vi "Write HttpRequestMessage.vi"(8 "error in (no error)":errorcluster, 10 "LabVIEWHTTPClient_NET.lvlib:HttpRequestMessage.lvclass":refnum<class "HttpRequestMessage.lvclass">, 11 "HttpResponseMessage in":refnum<class "HttpResponseMessage.lvclass">) -> (0 "error out":errorcluster, 3 "HttpResponseMessage out":refnum<class "HttpResponseMessage.lvclass">)   [LabVIEW 2018, in "LabVIEWHTTPClient_NET.lvlib" / "HttpResponseMessage.lvclass"]
uses:
  HttpResponseMessage.lvclass
  HttpRequestMessage/HttpRequestMessage.lvclass
  HttpResponseMessage.lvclass/HttpResponseMessage.ctl
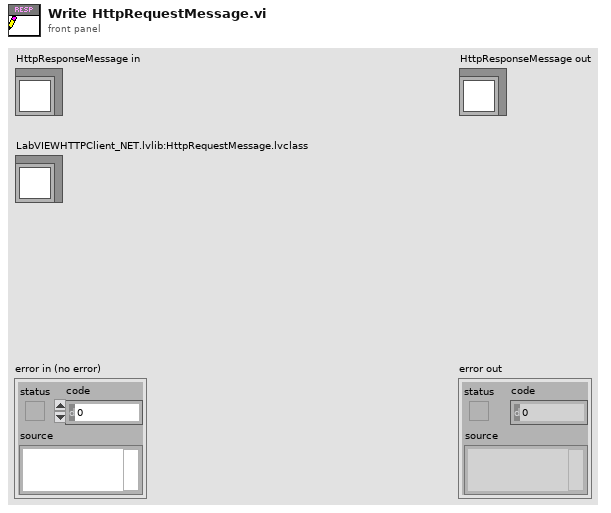
[diagram p1: front panel]
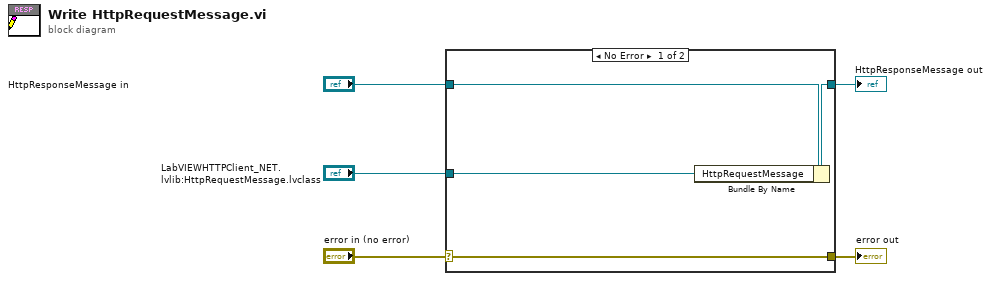
[diagram p0: block diagram]
diagram:
  n1 = case shown="No Error" "error in (no error)" {
    selector: "error in (no error)" -> [w9 w10]
    tunnel: [w9 w10] -> w4
    tunnel: [w7 w11] -> w2
    tunnel: "HttpResponseMessage in" -> [w8 w11]
    tunnel: "LabVIEWHTTPClient_NET.lvlib:HttpRequestMessage.lvclass" -> [w6 _]
    frame No Error {
      n2 = Bundle By Name(cluster=w8, "HttpRequestMessage"=w6) -> (w7:refnum<class "HttpResponseMessage.lvclass">)
    }
    frame Error {
    }
  }
  "error out" <- w4
  "HttpResponseMessage out" <- w2
